vi "setUp.vi"(8 "error in (no error)":errorcluster, 11 "reference in":refnum<class "ListImp_Functional.lvclass">) -> (0 "error out":errorcluster, 3 "reference in":refnum<class "ListImp_Functional.lvclass">)   [LabVIEW 2009, in "ListImp_Functional.lvclass"]
doc: "setUp runs prior to the test method during test execution. Use this method to initialize any object data required by your tests."
uses:
  ListImp_Functional.lvclass
  ListImp_Functional.lvclass/ListImp_Functional.ctl
  <vilib>/addons/_JKI Toolkits/VI Tester/TestCase.llb/TestCase.lvclass
  source/Lists/List/List.lvclass
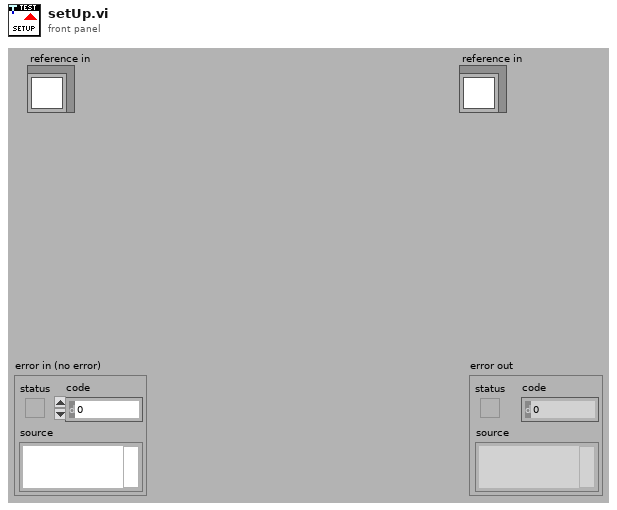
[diagram p1: front panel]
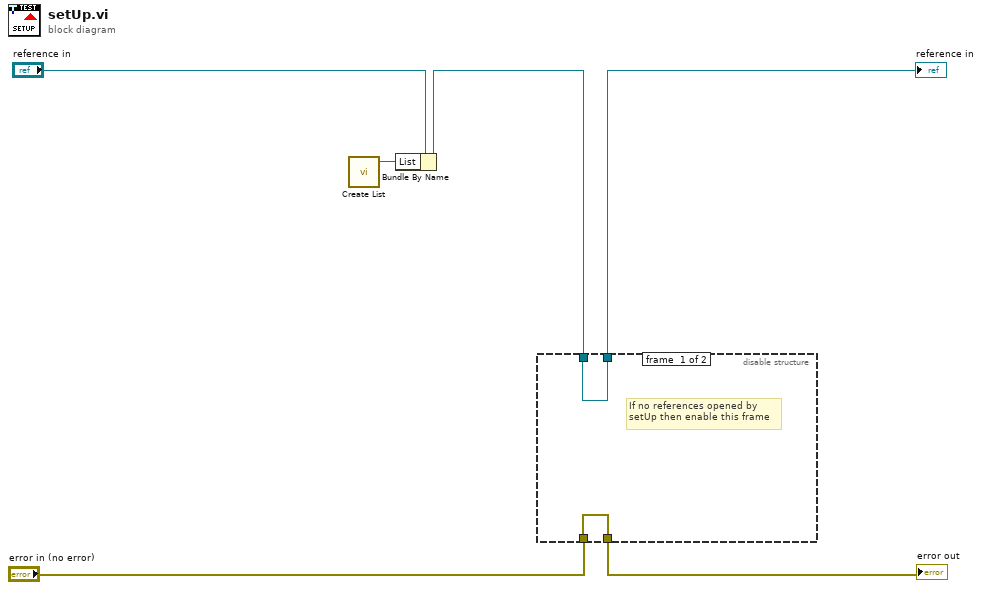
[diagram p0: block diagram]
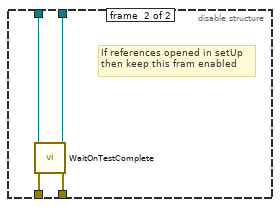
[diagram p2: hidden frame]
diagram:
  n1 = call "Create List.vi"() -> ("List out"=w1:refnum<class "List.lvclass">)  [unwired: 10 in, 1 out]
  n2 = Bundle By Name(cluster="reference in", "List"=w1) -> (w2:refnum<class "ListImp_Functional.lvclass">)
  n3 = disable-structure shown="Enabled" {
    disable-tunnel: w2 -> [w8 w12]
    disable-tunnel: [w8 w11] -> w3
    disable-tunnel: "error in (no error)" -> [w7 w10]
    disable-tunnel: [w7 w9] -> w5
    frame #0 {
      # "If no references opened by\nsetUp then enable this frame"
    }
    frame #1 {
      # "If references opened in setUp\nthen keep this fram enabled"
      n4 = call <vilib>:"WaitOnTestComplete.vi"("error in (no error)"=w10, "TestCase in"=w12) -> ("error out"=w9:errorcluster, "TestCase out"=w11:refnum<class "ListImp_Functional.lvclass">)  [unwired: 8 in]
    }
  }
  "error out" <- w5
  "reference in" <- w3
